vi "meter-1.vi"() -> ()   [LabVIEW 2010]
uses:
  VarableID.ctl
panel:
  out "Data1":string
  in  "视在功率":bool
  in  "功率因数":bool
  in  "电压":bool
  in  "电流":bool
  in  "baud rate":u32=2400 caption="波特率"
  in  "退出系统":bool
  in  "软件使用说明":bool
  out "测量变量显示":dbl[](graph)
  in  "启动采集":bool=TRUE
  in  "Port":refnum<visa-resource-name>="COM1" caption="端口号"
  # "智能电表信息采集系统"
  # "端口参数设置"
  # "信号采集选项"
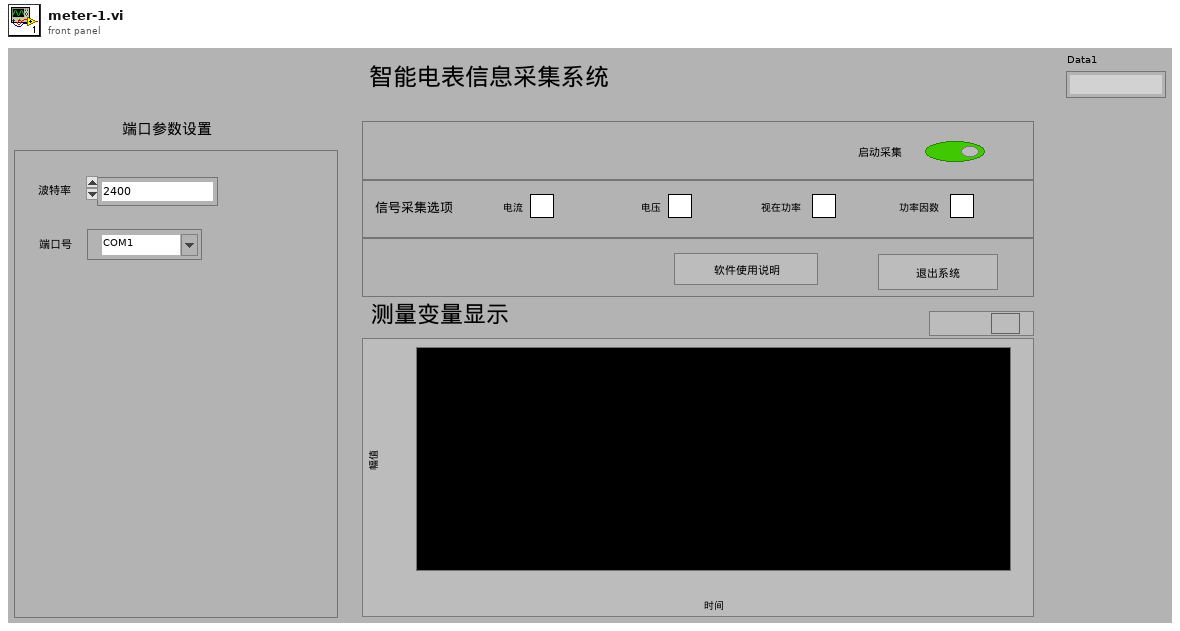
[diagram p1: front panel]
types:
  T1 = typedef "VarableID.ctl" = enum16{"current", "voltage", "power", "PF"}
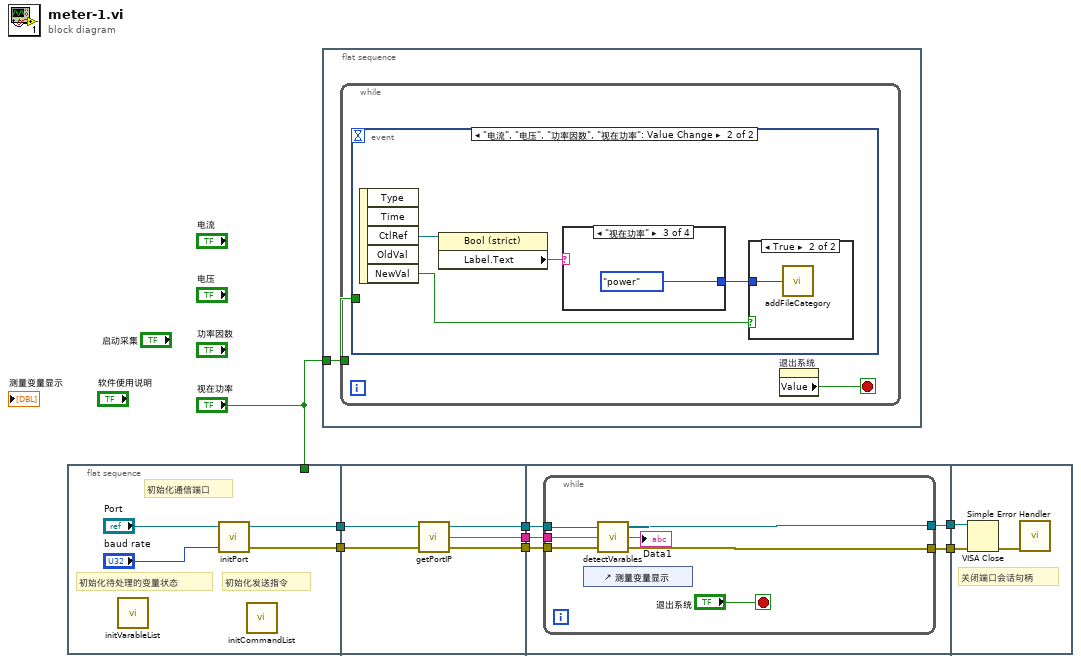
[diagram p0: block diagram]
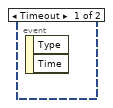
[diagram p2: hidden frame]
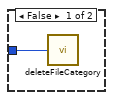
[diagram p3: hidden frame]
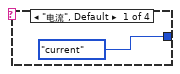
[diagram p4: hidden frame]
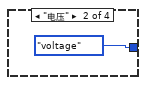
[diagram p5: hidden frame]
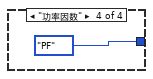
[diagram p6: hidden frame]
diagram:
  n1 = flat-sequence {
    tunnel: [w11] -> w4
    tunnel: "视在功率" -> [_]
    tunnel: [w9] -> w2
    tunnel: [w13] -> w5
    tunnel: w4 -> [w16]
    tunnel: [w15] -> w3
    tunnel: w2 -> [w17]
    tunnel: [w14] -> w1
    tunnel: w5 -> [w21]
    tunnel: w3 -> [w22]
    tunnel: [w20] -> w8
    tunnel: [w19] -> w7
    tunnel: w1 -> [w18]
    tunnel: w8 -> [w31]
    tunnel: w7 -> [w30]
    frame #0 {
      # "初始化发送指令"
      # "初始化通信端口"
      # "初始化待处理的变量状态"
      n2 = call "initVarableList.vi"() -> ()  [unwired: 12 in]
      n3 = call "initPort.vi"("baud rate"="baud rate", "VISA resource name"="Port") -> ("error out"=w9:errorcluster, "reference out"=w11:refnum<visa-resource-name>)  [unwired: 2 in]
      n4 = call "initCommandList.vi"() -> ()  [unwired: 12 in]
    }
    frame #1 {
      n5 = call "getPortIP.vi"("error in (no error)"=w17, "VISA resource name"=w16) -> ("error out"=w13:errorcluster, "portIP"=w14:string, "VISA resource name 2"=w15:refnum<visa-resource-name>)  [unwired: 1 in]
    }
    frame #2 {
      n6 = while {
        tunnel: w22 -> [w28]
        tunnel: w21 -> [w26]
        tunnel: [w27] -> w20
        tunnel: [w23] -> w19
        tunnel: w18 -> [w25]
        stop <- "退出系统" stop-if-true
        n7 = control-ref of="测量变量显示"() -> ()  [unwired: 1 out]
        n8 = call "detectVarables.vi"("error in (no error)"=w26, "PortIP"=w25, "VISA resource name"=w28) -> ("error out"=w23:errorcluster, "Data"=→"Data1":string, "VISA resource name 2"=w27:refnum<visa-resource-name>)
      }
    }
    frame #3 {
      # "关闭端口会话句柄"
      n9 = VISA Close(VISA resource name=w31, error in (no error)=w30) -> (error out=w32:errorcluster)
      n10 = call <vilib>:"Simple Error Handler.vi"("error in (no error)"=w32) -> ()  [unwired: 1 in, 8 out]
    }
  }
  n11 = flat-sequence {
    tunnel: "视在功率" -> [w33]
    frame #0 {
      n12 = while {
        tunnel: w33 -> [w35]
        stop <- w34 stop-if-true
        n13 = event shown="[1] \"电流\", \"电压\", \"功率因数\", \"视在功率\": Value Change" {
          selector: _ -> [_ _]
          dyn-events: _ -> [_ _]
          timeout: _ -> [_ _]
          tunnel: w35 -> [_ _]
          event Timeout {
            n14 = event-data() -> ()  [unwired: 1 in, 2 out]
          }
          event "电流", "电压", "功率因数", "视在功率": Value Change {
            n15 = event-data() -> ("CtlRef"=w36:refnum<vi>, "NewVal"=w37:bool)  [unwired: 1 in, 3 out]
            n16 = property class="Bool (strict)"(reference=w36) -> ("Label.Text"=w39:string)  [unwired: 1 in, 2 out]
            n17 = case shown="\"视在功率\"" w39 {
              tunnel: [VarableID."current" ("VarableID") VarableID."voltage" ("VarableID") VarableID."power" ("VarableID") VarableID."PF" ("VarableID")] -> w38
              frame "电流", Default {
              }
              frame "电压" {
              }
              frame "视在功率" {
              }
              frame "功率因数" {
              }
            }
            n18 = case shown="True" w37 {
              tunnel: w38 -> [w40 w41]
              frame False {
                n19 = call "deleteFileCategory.vi"("VarableID"=w40) -> ()  [unwired: 1 in]
              }
              frame True {
                n20 = call "addFileCategory.vi"("VarableID"=w41) -> ()  [unwired: 1 in]
              }
            }
          }
        }
        n21 = property on="退出系统" class="Bool (strict)"() -> ("Value"=w34:bool)  [unwired: 2 in, 2 out]
      }
    }
  }
